vi "Create Zone.vi"(5 "Zone in":refnum<class "Zone.lvclass">, 8 "error in (no error)":errorcluster, 11 "Zone Name":string) -> (0 "error out":errorcluster, 3 "Zone out":refnum<class "Zone.lvclass">)   [LabVIEW 2017, in "Zone.lvclass"]
uses:
  Zone.lvclass
  Zone.lvclass/Zone.ctl
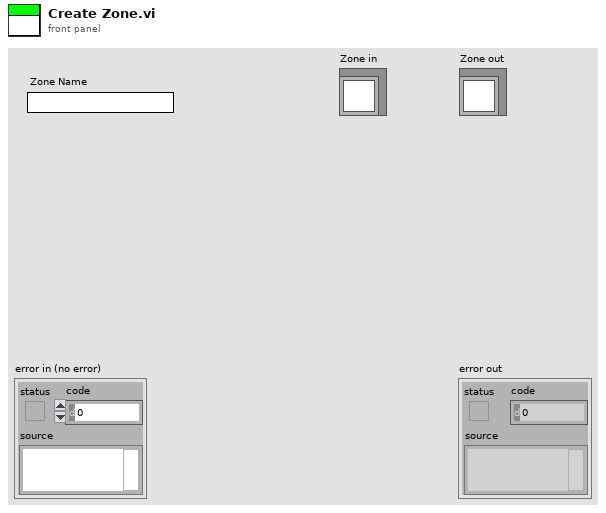
[diagram p1: front panel]
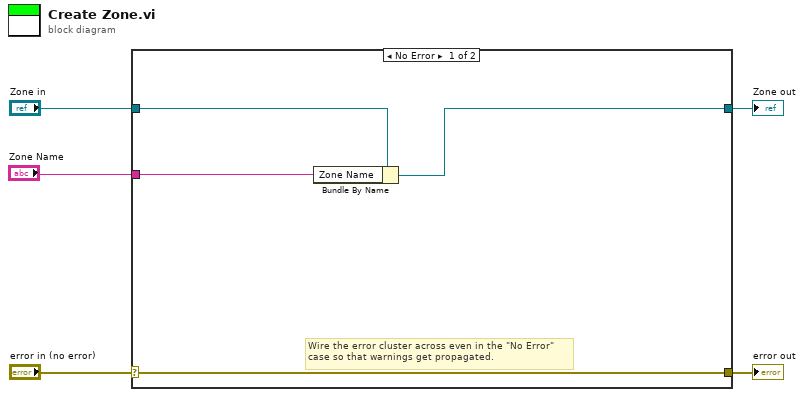
[diagram p0: block diagram]
diagram:
  n1 = case shown="No Error" "error in (no error)" {
    selector: "error in (no error)" -> [w9 w11]
    tunnel: [w9 w11] -> w4
    tunnel: [w6 w10] -> w2
    tunnel: "Zone in" -> [w7 w10]
    tunnel: "Zone Name" -> [w8 _]
    frame No Error {
      # "Wire the error cluster across even in the \"No Error\"\ncase so that warnings get propagated."
      n2 = Bundle By Name(cluster=w7, "Zone Name"=w8) -> (w6:refnum<class "Zone.lvclass">)
    }
    frame Error {
    }
  }
  "error out" <- w4
  "Zone out" <- w2
